vi "Get Waveform Quadrature.vi"(8 "error in (no error)":errorcluster, 11 "Reference in":waveform(dbl)) -> (0 "error out":errorcluster, 2 "Reference Channel":string, 3 "Reference out":waveform(dbl))   [LabVIEW 2019, in "Instrument.Lockin.lvlib" / "Instrument.DAQ.lvclass"]
uses:
  Instrument.DAQ.lvclass
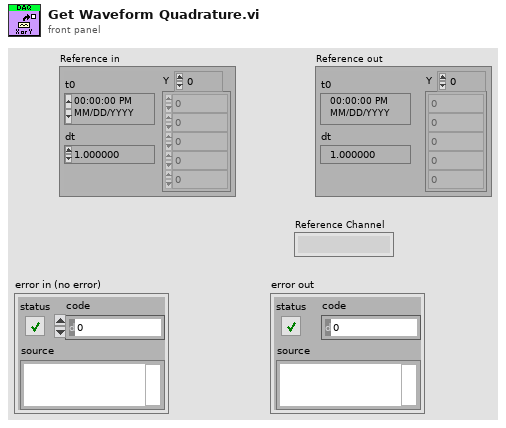
[diagram p1: front panel]
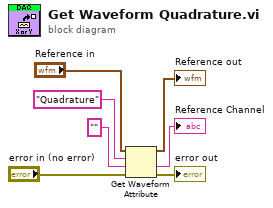
[diagram p0: block diagram]
diagram:
  n1 = Get Waveform Attribute(4:"error in (no error)", 5:"", 6:"Quadrature" ("name"), 7:"Reference in") -> (0:→"error out":errorcluster, 1:→"Reference Channel":string, 3:→"Reference out":waveform(dbl))  [unwired: 1 out]
